vi "SetPreset.vi"(6 "Legacy (f)?":bool, 8 "error in (no error)":errorcluster) -> (0 "error out":errorcluster)   [LabVIEW 2011]
uses:
  DUTport.ctl
  MeasMode.ctl
  HW Averaging.ctl
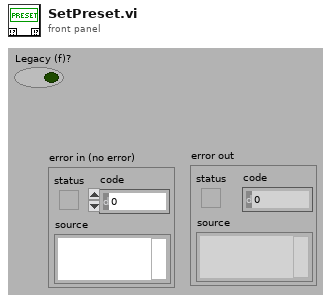
[diagram p1: front panel]
types:
  T1 = typedef "DUTport.ctl" = enum16{"Port 1", "Port 2"}
  T2 = typedef "MeasMode.ctl" = u16
  T3 = typedef "HW Averaging.ctl" = u16
  T4 = typedef "Test Set Definition.ctl" = cluster{"General":cluster{"ID":u32, "Model":string, "Dual Port?":bool, "Options":string, "Options":cluster{"E":bool, "K":bool, "H":bool, "W":bool, "F":bool}, "Cal File":path}, "Receiver":cluster{"Fstart, MHz":dbl, "Fstop MHz":dbl, "Fstep MHz":dbl, "IF, MHz":dbl}, "RX Band":cluster{"Fstart, MHz":dbl, "Fstop MHz":dbl}, "TX 1":cluster{"Fstart, MHz":dbl, "Fstop MHz":dbl, "Pmax, dBm":dbl, "Pstep, dB":dbl}, "TX 2":cluster{"Fstart, MHz":dbl, "Fstop MHz":dbl, "Pmax, dBm":dbl, "Pstep, dB":dbl}, "Low-side?":bool}
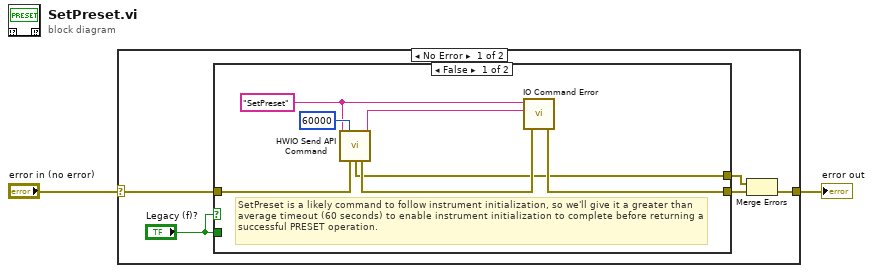
[diagram p0: block diagram]
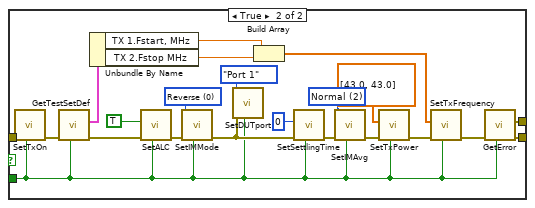
[diagram p2: hidden frame]
diagram:
  n1 = case shown="No Error" "error in (no error)" {
    selector: "error in (no error)" -> [w7 w37]
    tunnel: [w3 w37] -> w2
    frame No Error {
      n2 = case shown="False" "Legacy (f)?" {
        tunnel: "Legacy (f)?" -> [_ w16]
        tunnel: w7 -> [w14 w22]
        tunnel: [w10 w20] -> w4
        tunnel: [w8 w21] -> w5
        frame False {
          w12 = "SetPreset"
          # "SetPreset is a likely command to follow instrument initialization, so we'll give it a greater than average timeout (60 seconds) to enable instrument initialization to complete before returning a successful PRESET operation."
          n3 = call "HWIO Send API Command.vi"("Action"=w12, "Timeout ms (5000)"=60000 ("Command Timeout (ms)"), "error in (no error)"=w14) -> ("Action out"=w11:string, "HWError"=w8:errorcluster, "error out"=w9:errorcluster)  [unwired: 5 in, 5 out]
          n4 = call "IO Command Error.vi"("error in (no error)"=w9, "Command Returned (\"\")"=w11, "Command Sent (\"\")"=w12) -> ("error out"=w10:errorcluster)  [unwired: 4 out]
        }
        frame True {
          w18 = T2 0 items=["Reverse", "Forward", "Auxiliary"] ("SetIMMode")
          w29 = T3 2 items=["None", "Minimum", "Normal", "High", "Maximum"] ("SetIMAvg")
          n5 = call "SetTxOn.vi"("Legacy (f)?"=w16, "error in (no error)"=w22) -> ("error out"=w36:errorcluster)  [unwired: 8 in, 1 out]
          n6 = call "GetTestSetDef.vi"("Legacy (f)?"=w16, "error in (no error)"=w36) -> ("error out"=w31:errorcluster, "TestSetDef"=w35:T4)  [unwired: 8 in]
          n7 = Unbundle By Name(w35) -> ("TX 1.Fstart, MHz"=w34:dbl, "TX 2.Fstop MHz"=w33:dbl)
          n8 = call "SetALC.vi"("Legacy (f)?"=w16, "error in (no error)"=w31, "ALC"=TRUE) -> ("error out"=w19:errorcluster)  [unwired: 8 in]
          n9 = call "SetIMMode.vi"("Legacy (f)?"=w16, "error in (no error)"=w19, "SetIMMode"=w18) -> ("error out"=w17:errorcluster)  [unwired: 8 in]
          n10 = call "SetDUTport.vi"("Legacy (f)?"=w16, "error in (no error)"=w17, "SetDUTport"=DUTport."Port 1") -> ()  [unwired: 8 in, 1 out]
          n11 = Build Array(w34, w33) -> (w24:dbl[])
          n12 = call "SetSettlingTime.vi"("Legacy (f)?"=w16, "error in (no error)"=w17, "SettlingTime"=u32 0) -> ("error out"=w28:errorcluster)  [unwired: 8 in]
          n13 = call "SetIMAvg.vi"("Legacy (f)?"=w16, "error in (no error)"=w28, "SetIMAvg"=w29) -> ("error out"=w27:errorcluster)  [unwired: 8 in]
          n14 = call "SetTxPower.vi"("Legacy (f)?"=w16, "error in (no error)"=w27, "TxPower"=dbl[] [43.0, 43.0]) -> ("error out"=w25:errorcluster)  [unwired: 8 in]
          n15 = call "SetTxFrequency.vi"("Legacy (f)?"=w16, "error in (no error)"=w25, "TxFrequencies"=w24) -> ("error out"=w23:errorcluster)  [unwired: 8 in]
          n16 = call "GetError.vi"("Legacy (f)?"=w16, "error in (no error)"=w23) -> ("error out"=w20:errorcluster, "HW Error"=w21:errorcluster)  [unwired: 8 in]
        }
      }
      n17 = Merge Errors(w5, w4) -> (w3:errorcluster)
    }
    frame Error {
    }
  }
  "error out" <- w2
